vi "Read Config Unitest.vi"(8 "error in (no error)":errorcluster, 11 "main ref":T1) -> (0 "error out":errorcluster)   [LabVIEW 2025]
uses:
  v06/controls/LAB-IQ UI Data.ctl
  Traction Loop/Traction Receipe Enum.ctl
  Config file  FGV Unitest enum.ctl
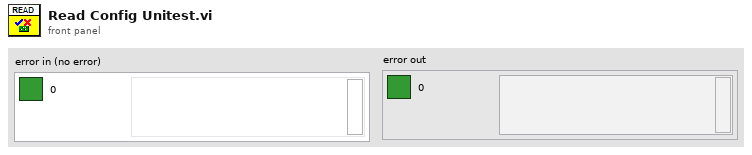
[diagram p1: front panel]
types:
  T1 = typedef "LAB-IQ UI Data.ctl" = cluster{"Main Home Screen":cluster{"GUI":refnum<vi>, "Platform Settings":refnum<vi>, "Configure":refnum<vi>, "Home":refnum<vi>, "EXIT":refnum<vi>, "service 2":refnum<vi>, "MainPage":refnum<vi>, "Analysis":refnum<vi>}, "Platform Settings":cluster{"mm/s  Surge":refnum<vi>, "Drive Error":refnum<vi>, "Disable Axis Jog Soft Limits":refnum<vi>, "mm/s  Sway":refnum<vi>, "Sway and Surge COM Status":refnum<vi>, "Heave COM Status":refnum<vi>, "Enable Platform":refnum<vi>, "Surge Forward Main":refnum<vi>, "Sway Right Main":refnum<vi>, "Sway Left Main":refnum<vi>, "Heave Down Main":refnum<vi>, "Heave Up main":refnum<vi>, "mm/s Heave":refnum<vi>, "mm/sec":refnum<vi>, "mm":refnum<vi>, "Surge Backward Main":refnum<vi>}, "Analysis Screen":cluster{"Analysis Home":refnum<vi>, "Surface Analysis":refnum<vi>, "Imaging":refnum<vi>, "Image Analysis":refnum<vi>, "Post Analysis":refnum<vi>}, "Config Screen":cluster{"Select Load Head":refnum<vi>, "Notes :":refnum<vi>, "FILE":refnum<vi>, "Sample ID :":refnum<vi>, "Operator ID :":refnum<vi>, "Operator Name :":refnum<vi>, "Auto":refnum<vi>}, "Motion Module":cluster{"zNL":refnum<vi>, "NL disp":refnum<vi>, "Rotary Tab":refnum<vi>, "Motion Direction:  3":refnum<vi>, "E.Velocity 2":refnum<vi>, "e.v/ssr 2":refnum<vi>, "Enter Fixed E.Velocity 2":refnum<vi>, "Enter Final SRR 2":refnum<vi>, "Enter initial SRR 2":refnum<vi>, "Enter Fixed SRR 2":refnum<vi>, "Enter the Final E.Velocity (m/s) 2":refnum<vi>, "Enter initial E.Velocity (m/s) 2":refnum<vi>, "Final Speed (RPM) 3":refnum<vi>, "Initial Speed (RPM) 2":refnum<vi>, "Enter the Final Velocity (m/s) 3":refnum<vi>, "Enter initial Velocity (m/s)  3":refnum<vi>, "Ramp Up 2":refnum<vi>, "TEST SELECTION":refnum<vi>, "SPEED SELECTION : ":refnum<vi>, "Angular Oscillation Set":refnum<vi>, "Traction":refnum<vi>, "Step Speed":refnum<vi>, "StepTable For Load-Speed":refnum<vi>, "StepTable For Speed":refnum<vi>, "Surge Forward MM":refnum<vi>, "Surge Backward MM":refnum<vi>, "M3 Image":refnum<vi>, "String 39":refnum<vi>, "Sway Left MM":refnum<vi>, "Sway Right MM":refnum<vi>, "Disable Axis Jog Soft Limits":refnum<vi>, "mm":refnum<vi>, "Heave Down MM":refnum<vi>, "Heave Up MM":refnum<vi>, "Wear Track Diameter (mm)":refnum<vi>, "Set WTD":refnum<vi>, "HomeScratch":refnum<vi>, "HomeRot":refnum<vi>, "PlaceModule":refnum<vi>, "Enter the Angle (Deg)":refnum<vi>, "Enter the Frequency (Hz)":refnum<vi>, "Motion Mode:":refnum<vi>, "LR Sway":refnum<vi>, "Rot Hor":refnum<vi>, "Scratch":refnum<vi>, "LR Cam":refnum<vi>, "MMBack":refnum<vi>, "MMNext":refnum<vi>, "Rot Ver":refnum<vi>, "Rotary Module Selection":refnum<vi>, "calculate rotary":refnum<vi>, "SPEED SELECTION : rotary":refnum<vi>, "Import 2":refnum<vi>, "Save 2":refnum<vi>, "File Path :  2":refnum<vi>, "String 45":refnum<vi>, "StepTable For Speed 3":refnum<vi>, "Enter the Speed(mm/sec)":refnum<vi>, "Enter the Speed(RPM)":refnum<vi>, "Enter Scratch Speed (mm/s):":refnum<vi>, "SwaySpeed Set":refnum<vi>, "Scartch Offset":refnum<vi>, "Motion type:":refnum<vi>, "HomeScratch 2":refnum<vi>, "Enter Scratch length (mm):":refnum<vi>, "Wear Track Diameter":refnum<vi>, "Rotary Speed Exced":refnum<vi>, "Scratch Mode":refnum<vi>, "No of Scratch":refnum<vi>}, "Environmental control":cluster{"Humidity  Status  3":refnum<vi>, "Low Temp  Status  2":refnum<vi>, "TK4 status 2":refnum<vi>, "Stage Temperature":refnum<vi>, "Sample Temperature":refnum<vi>, "Humidity (Amb)":refnum<vi>, "Clear List":refnum<vi>, "Add to list":refnum<vi>, "Wear":refnum<vi>, "Vibration":refnum<vi>, "Humidity (Chamber)":refnum<vi>, "Temperature (Chamber)":refnum<vi>, "ECR ":refnum<vi>, "Temperature (Amb)":refnum<vi>, "Microphone":refnum<vi>, "Acoustic Emission 3":refnum<vi>, "SNext":refnum<vi>, "APBack":refnum<vi>, "Enter the Temperature (°C):":refnum<vi>, "Enter the Stage \nTemperature (°C):":refnum<vi>, "Enter the Humidity (%Rh):":refnum<vi>, "Low Temp":refnum<vi>, "High Temp":refnum<vi>, "Humidity":refnum<vi>, "Sensors Picked":refnum<vi>}, "About Screen":cluster{"Password":refnum<vi>, "Home Service":refnum<vi>, "Advanced Setting":refnum<vi>, "About Tab":refnum<vi>, "ECR Port:":refnum<vi>, "Ramp Port:":refnum<vi>, "Installation/Replacement completed":refnum<vi>, "Loahead":refnum<vi>, "Heave and Surge COM Port:":refnum<vi>, "Sway COM Port:":refnum<vi>, "Temp Modbus:":refnum<vi>, "Humidity Port:":refnum<vi>, "Edit Gain Constants":refnum<vi>, "Save Gain Constants":refnum<vi>}, "Main Screen":cluster{"Main Screen Tab":refnum<vi>, "Angle and Frequency":refnum<vi>, "Stroke (mm)":refnum<vi>, "Angle (Deg)":refnum<vi>, "Main Speed Tab":refnum<vi>, "MTM MOTOR DISPLAY":refnum<vi>, "Disc Speed (m/sec)":refnum<vi>, "Ball Speed (m/sec)":refnum<vi>, "Disc Speed (RPM)":refnum<vi>, "Ball Speed (RPM)":refnum<vi>, "SPEED TAB":refnum<vi>, "Speed (m/sec)":refnum<vi>, "Set Speed (m/sec)":refnum<vi>, "Speed (RPM)":refnum<vi>, "Set Speed":refnum<vi>, "Time Tab":refnum<vi>, "Time ( HH:MM:SS ) 2":refnum<vi>, "Test Duration":refnum<vi>, "Test Duration 4":refnum<vi>, "TEST CYCLE":refnum<vi>, "TOTAL CYCLES":refnum<vi>, "Set Load (N)":refnum<vi>, "Temp Tabs":refnum<vi>, "Heater":refnum<vi>, "TK4 status":refnum<vi>, "ChamberTemp":refnum<vi>, "SetTmp":refnum<vi>, "Controller  Status":refnum<vi>, "ChamberTemp 2":refnum<vi>, "SetTmp 2":refnum<vi>, "Controller  Status 2":refnum<vi>, "ChamberTemp 3":refnum<vi>, "SetTmp 3":refnum<vi>, "Cooling":refnum<vi>, "Load Communication":refnum<vi>, "Ambient \nTemperature":refnum<vi>, "HumCOMStatus":refnum<vi>, "Ambient\n Humidity":refnum<vi>, "Freq (Hz)":refnum<vi>, "Load En":refnum<vi>, "NLt":refnum<vi>, "zNL 2":refnum<vi>, "Humidity On":refnum<vi>, "humidity disp":refnum<vi>, "Set Humidity":refnum<vi>, "NL disp 2":refnum<vi>, "Humidity On 2":refnum<vi>, "humidity disp 2":refnum<vi>, "Set Humidity 2":refnum<vi>, "NL disp 3":refnum<vi>, "AppLoadSeq scratch":refnum<vi>, "Stop Scratch":refnum<vi>, "ClrLog":refnum<vi>, "Trip Log":refnum<vi>, "STOP":refnum<vi>, "Start Test":refnum<vi>, "Test status":refnum<vi>, "AR Led":refnum<vi>, "Data":refnum<vi>, "Health":refnum<vi>, "Sway COM Status":refnum<vi>, "Heave COM Status":refnum<vi>, "Grp Tab":refnum<vi>, "Sub Graph":refnum<vi>, "SD (mm)":refnum<vi>, "Siliding distance Reset Graph":refnum<vi>, "SDGp":refnum<vi>, "Humidity Reset Graph":refnum<vi>, "HumrGp":refnum<vi>, "Acoustic Emission (mV)":refnum<vi>, "Aqucostic Reset Graph":refnum<vi>, "gACQUOS":refnum<vi>, "ECR RESET":refnum<vi>, "ECR":refnum<vi>, "Temperature Reset":refnum<vi>, "Acoustic Emission (mV) 2":refnum<vi>, "Aqucostic Reset Graph 2":refnum<vi>, "gACQUOS 2":refnum<vi>, "ECR RESET 2":refnum<vi>, "ECR 2":refnum<vi>, "Temperature Reset 2":refnum<vi>, "Temperature (deg c)":refnum<vi>, "Speed Reset Graph":refnum<vi>, "Speed Tab":refnum<vi>, "MTM DISC  SPEED":refnum<vi>, "MTM BALL SPEED":refnum<vi>, "speed mm/sec":refnum<vi>, "Hymidity":refnum<vi>, "Humidity Disable trip":refnum<vi>, "CoF Trip  2":refnum<vi>, "Depth Trip":refnum<vi>, "Weart Deapth":refnum<vi>, "Depth Reset Graph":refnum<vi>, "Weart":refnum<vi>, "Depthz":refnum<vi>, "Depth (µm)":refnum<vi>, "WearGp":refnum<vi>, "NL Trip 2":refnum<vi>, "Load pid":refnum<vi>, "Load Disable Trip":refnum<vi>, "Load Reset Graph":refnum<vi>, "NL Display 4":refnum<vi>, "Main Chart 3":refnum<vi>, "BACK":refnum<vi>, "Depth Trip 2":refnum<vi>, "COF TRIP ":refnum<vi>, "Friction Force (N)":refnum<vi>, "FF Reset Graph":refnum<vi>, "FF Disable Trip":refnum<vi>, "FF TRIP":refnum<vi>, "COF Disable Trip":refnum<vi>, "COF Reset Graph":refnum<vi>, "Start Test Temp":refnum<vi>, "zFF":refnum<vi>, "Friction Force (N) Graph":refnum<vi>, "Coefficient of Friction":refnum<vi>, "Scratch Start Test":refnum<vi>, "FF Tab":refnum<vi>, "Cyclic Friction Force (N)":refnum<vi>, "CZ FF":refnum<vi>, "Cyclic Friction Force (N) Graph":refnum<vi>, "Cyclic Coefficient of Friction":refnum<vi>, "Cyclic FF TRIP":refnum<vi>, "Cyclic FF Disable Trip":refnum<vi>, "cyclic COF Disable Trip":refnum<vi>, "cyclic COF TRIP":refnum<vi>, "cyclic COF Reset Graph":refnum<vi>, "Cyclic FF Reset Graph":refnum<vi>, "Test Trip":refnum<vi>, "Multi Scratch Pass":refnum<vi>, "Scratch Start Recording":refnum<vi>, "Coefficient of Friction 2":refnum<vi>, "Acoustic Emission":refnum<vi>, "Friction Force (N) 2":refnum<vi>, "Depth (Microns)":refnum<vi>, "Normal Load ( N )":refnum<vi>}, "Loading":cluster{"Indentation":refnum<vi>, "Reference Sample":refnum<vi>, "Load Cell Communication Slide":refnum<vi>, "com 3":refnum<vi>, "com":refnum<vi>, "DecaForce COM Status":refnum<vi>, "Update":refnum<vi>, "Clear 3":refnum<vi>, "seq":refnum<vi>, "Stribeck table":refnum<vi>, "Stribeck Table  For loading":refnum<vi>, "Loading Mode":refnum<vi>, "Enter the Final Load (N)":refnum<vi>, "Enter the CoF Trip":refnum<vi>, "Enter the Friction Force Trip":refnum<vi>, "Enter the Normal load Trip":refnum<vi>, "Enter the Load  (N)":refnum<vi>, "KiloForce":refnum<vi>, "DecaForce ":refnum<vi>, "MicroForce":refnum<vi>, "LHBack":refnum<vi>, "LHNext":refnum<vi>, "Enter the Loading Rate (N/min)":refnum<vi>, "Message":refnum<vi>, "Warning 2":refnum<vi>, "SSP 0.75":refnum<vi>, "SSP 0.5":refnum<vi>, "SSP 0.3":refnum<vi>, "Warning":refnum<vi>, "gui GIF":refnum<vi>, "Communication is established":refnum<vi>, "AppLoad 4":refnum<vi>, "Multipoint":refnum<vi>, "Load Selection":refnum<vi>}, "PID":cluster{"Ramp":refnum<vi>, "Vertical load (N)":refnum<vi>, "apply load":refnum<vi>, "apply load 2":refnum<vi>, "Enter ByPass Load":refnum<vi>, "Bypass Load":refnum<vi>, "gFF Rot":refnum<vi>}, "Config Parameters":cluster{"Tab Control 3":refnum<vi>, "Tab Control 19":refnum<vi>, "SAMPLES":refnum<vi>, "Re-initilaize":refnum<vi>, "Filter ON/OFF":refnum<vi>, "TracHomeSurgeOffsetCounts 10MM":refnum<vi>, "TracHomeSwayOffsetCounts 10MM":refnum<vi>, "Acoustic Emission:":refnum<vi>, "Apply Filter (FF)":refnum<vi>, "Filter% 2":refnum<vi>, "Apply Filter (Load)":refnum<vi>, "Filter% ":refnum<vi>, "Sway distance (mm)":refnum<vi>, "Surge distance (mm)":refnum<vi>, "DataSavingLoopDelay(ms)":refnum<vi>, "SAVE 2":refnum<vi>, "Enter Distance":refnum<vi>, "Sway Counts:":refnum<vi>, "Distance (mm): 3":refnum<vi>, "Surge Counts:":refnum<vi>, "Distance (mm): 2":refnum<vi>, "Distance (mm):":refnum<vi>, "Heave Counts:":refnum<vi>, "LRMHomeSurgeOffsetCounts":refnum<vi>, "LRMHomeSwayOffsetCounts":refnum<vi>, "TracHomeSurgeOffsetCounts 20MM":refnum<vi>, "TracHomeSwayOffsetCounts 20MM":refnum<vi>, "RotHomeSwayOffsetCounts":refnum<vi>, "RotHomeSurgeOffsetCounts":refnum<vi>, "Heave distance":refnum<vi>, "Zmm":refnum<vi>, "Heave Pulses/mm":refnum<vi>, "Surge Pulses/mm":refnum<vi>, "Sway Pulses/mm":refnum<vi>, "Heave Pitch":refnum<vi>, "Surge Pitch":refnum<vi>, "Sway Pitch":refnum<vi>, "Heave PPR":refnum<vi>, "Surge PPR":refnum<vi>, "Sway PPR":refnum<vi>, "Tab Control 5":refnum<vi>, "Tab Control 14":refnum<vi>, "Tab Control 26":refnum<vi>, "AE":refnum<vi>, "Heave Loop Delay":refnum<vi>, "Heave PID Speed":refnum<vi>, "Surge Jog Speed":refnum<vi>, "Heave Jog Speed":refnum<vi>, "Sway Loop Delay":refnum<vi>, "Sway PID Speed":refnum<vi>, "Sway Jog Speed":refnum<vi>, "DEPTH TRIP VALUE":refnum<vi>, "LOAD TRIP VALUE":refnum<vi>, "DEPTH TRIP   ENABLE":refnum<vi>, "LOAD TRIP  ENABLE":refnum<vi>, "CYCLIC FF TRIP VALUE":refnum<vi>, "FF TRIP VALUE":refnum<vi>, "CYCLIC CoF TRIP VALUE":refnum<vi>, "COF TRIP VALUE":refnum<vi>, "CYCLIC COF TRIP  ENABLE":refnum<vi>, "CYCLIC FF TRIP  ENABLE":refnum<vi>, "FF TRIP  ENABLE":refnum<vi>, "COF TRIP  ENABLE":refnum<vi>, "JOG TRIP LOAD VALUE (N)":refnum<vi>, "Rotary Vertical":refnum<vi>, "Traction":refnum<vi>, "Scratch":refnum<vi>, "LRM CAM":refnum<vi>, "Sway LRM":refnum<vi>, "Rotary Horizontal":refnum<vi>, "SURGE SPEED":refnum<vi>, "SURGE BACKWARD COUNT":refnum<vi>, "SURGE FORWARD COUNT":refnum<vi>, "Start Button":refnum<vi>}, "Loading Com Port":cluster{"ClearAll":refnum<vi>, "Mz(Nm)":refnum<vi>, "My(Nm)":refnum<vi>, "Mx(Nm)":refnum<vi>, "Save Dwell":refnum<vi>, "Acq Delay (ms)":refnum<vi>, "Burst Delay (ms)":refnum<vi>, "model":refnum<vi>, "SN":refnum<vi>, "FFx(N)":refnum<vi>, "Sensor IP":refnum<vi>, "Port":refnum<vi>, "FFy(N)":refnum<vi>, "Load(N)":refnum<vi>, "delete Handle":refnum<vi>, "Create Handle":refnum<vi>, "ft_data":refnum<vi>, "ft_range":refnum<vi>, "ft_data 2":refnum<vi>, "stop 6":refnum<vi>, "running_flag":refnum<vi>, "ft_udp_handle":refnum<vi>, "get-data-return":refnum<vi>, "get-range-return":refnum<vi>, "zero-return":refnum<vi>, "filter-return":refnum<vi>, "initial-return":refnum<vi>, "deleteHandle-result":refnum<vi>, "Load Cell Temp":refnum<vi>, "Load Cell":refnum<vi>, "ZeroAll":refnum<vi>, "FORCE (N)":refnum<vi>, "TORQUE (N-m)":refnum<vi>, "Load Cell Link":refnum<vi>}, "Heave AND Surge":cluster{"SURGE POSE":refnum<vi>, "error out Read":refnum<vi>, "HEAVE POSE":refnum<vi>, "State":refnum<vi>, "Homed":refnum<vi>, "Sequence ID":refnum<vi>, "error out Write":refnum<vi>, "faultCode":refnum<vi>, "Ack ID":refnum<vi>, "SPEED":refnum<vi>, "Distance":refnum<vi>, "Mode Command":refnum<vi>, "Heave and Surge Read":refnum<vi>, "Read Heave Temp":refnum<vi>, "Spare 15":refnum<vi>, "Spare 14":refnum<vi>, "Spare 13":refnum<vi>, "Spare 12":refnum<vi>, "Spare 11":refnum<vi>, "Spare 10":refnum<vi>, "Spare 9":refnum<vi>, "Spare 8":refnum<vi>, "Spare 7":refnum<vi>, "Spare 4":refnum<vi>, "Spare 3":refnum<vi>, "Spare 2":refnum<vi>, "Humidity":refnum<vi>, "Temp":refnum<vi>, "Node Id":refnum<vi>, "Spare 1":refnum<vi>, "SPARE 4":refnum<vi>, "SPARE 3":refnum<vi>, "SPARE 2":refnum<vi>, "SPARE 1":refnum<vi>, "fwMajor":refnum<vi>, "fwMinor":refnum<vi>, "Manual Write":refnum<vi>, "Heave and Surge Write":refnum<vi>, "SPARE 5":refnum<vi>, "Reserved ":refnum<vi>, "SPARE 8":refnum<vi>, "SPARE 6":refnum<vi>, "SPARE 7":refnum<vi>, "SPARE 17":refnum<vi>, "SPARE 16":refnum<vi>, "SPARE 15":refnum<vi>, "SPARE 14":refnum<vi>, "SPARE 13":refnum<vi>, "SPARE 12":refnum<vi>, "SPARE 11":refnum<vi>, "SPARE 10":refnum<vi>, "SPARE 9":refnum<vi>, "System UPTIME":refnum<vi>, "Missed Packets":refnum<vi>, "faultCode Surge Right":refnum<vi>, "faultCode Surge Left":refnum<vi>, "faultCode Heave":refnum<vi>, "UPLINK HEAVE":refnum<vi>, "DOWNLINK HEAVE":refnum<vi>}, "New PID LOGIC":cluster{"Fine Tune Zone":refnum<vi>, "PID SDelay":refnum<vi>, "Max_pos_limit":refnum<vi>, "Min_pos_limit":refnum<vi>, "i_limit":refnum<vi>, "pct_scale":refnum<vi>, "Deadband":refnum<vi>, "Kd":refnum<vi>, "Ki":refnum<vi>, "Kp":refnum<vi>, "Current Position":refnum<vi>, "Set Load":refnum<vi>, "Current Load":refnum<vi>, "Pulse delta":refnum<vi>, "Init Step":refnum<vi>, "Max Step Linit":refnum<vi>, "min_deadband_floor":refnum<vi>, "dynamic_spindle_noise_scalar":refnum<vi>, "min_finetune_floor":refnum<vi>, "filter_alpha":refnum<vi>, "PID":refnum<vi>}, "SWAY ":cluster{"fwMajor":refnum<vi>, "Homed":refnum<vi>, "Rotary POSE":refnum<vi>, "State":refnum<vi>, "SWAY POSE":refnum<vi>, "Ack ID":refnum<vi>, "faultCode":refnum<vi>, "Node Id":refnum<vi>, "fwMinor":refnum<vi>, "Spare 6":refnum<vi>, "Spare 5":refnum<vi>, "Spare 4":refnum<vi>, "Spare 3":refnum<vi>, "Spare 2":refnum<vi>, "Spare 1":refnum<vi>, "Spare 7":refnum<vi>, "SPARE  5":refnum<vi>, "error out Write  SWAY ":refnum<vi>, "error out Read SWAY ":refnum<vi>, "Manual Write SWAY ":refnum<vi>, "SWAY WRITE":refnum<vi>, "SPARE  4":refnum<vi>, "SPARE  3":refnum<vi>, "SPARE 2":refnum<vi>, "SPARE 1":refnum<vi>, "Spare 15":refnum<vi>, "Spare 14":refnum<vi>, "Spare 13":refnum<vi>, "Spare 12":refnum<vi>, "Spare 11":refnum<vi>, "Spare 9":refnum<vi>, "Spare 8":refnum<vi>, "SPEED":refnum<vi>, "Distance":refnum<vi>, "Mode Command":refnum<vi>, "Sequence ID":refnum<vi>, "SWAY READ":refnum<vi>, "Spare 10":refnum<vi>, "Read SWAY Temp":refnum<vi>, "faultCode Sway ":refnum<vi>, "Missed Packets":refnum<vi>, "System UPTIME sway":refnum<vi>, "SPARE 6":refnum<vi>, "SPARE 7":refnum<vi>, "SPARE 9":refnum<vi>, "SPARE 11":refnum<vi>, "SPARE 10":refnum<vi>, "SPARE 8":refnum<vi>, "SPARE 13":refnum<vi>, "SPARE 12":refnum<vi>, "SPARE 17":refnum<vi>, "SPARE 16":refnum<vi>, "SPARE 15":refnum<vi>, "SPARE 14":refnum<vi>, "Reserved":refnum<vi>, "faultCode Rotary":refnum<vi>, "UPLINK SWAY":refnum<vi>, "DOWNLINK SWAY":refnum<vi>}, "Analysis Screen":cluster{"Analysis Home":refnum<vi>, "Refresh 2":refnum<vi>, "MEAN 4":refnum<vi>, "SD 4":refnum<vi>, "VARIANCE 4":refnum<vi>, "MEAN  3":refnum<vi>, "SD  3":refnum<vi>, "VARIANCE  3":refnum<vi>, "MEAN 2":refnum<vi>, "SD  2":refnum<vi>, "VARIANCE 2":refnum<vi>, "MEAN":refnum<vi>, "SD":refnum<vi>, "VARIANCE":refnum<vi>, "File 4 Discription":refnum<vi>, "OPEN 4":refnum<vi>, "File Name 4":refnum<vi>, "OPEN 3":refnum<vi>, "File 3 Discription":refnum<vi>, "File Name 3":refnum<vi>, "Y-AXIS":refnum<vi>, "X-AXIS":refnum<vi>, "XY Graph":refnum<vi>, "File Name 2":refnum<vi>, "File Name 1":refnum<vi>, "OPEN 2":refnum<vi>, "OPEN 1":refnum<vi>, "File 1 Discription ":refnum<vi>, "File 2 Discription":refnum<vi>, "Export":refnum<vi>, "File Format":refnum<vi>}, "Traction":cluster{"faultCode Traction 2":refnum<vi>, "faultCode Traction 1":refnum<vi>, "Missed Packets":refnum<vi>, "System UPTIME Traction":refnum<vi>, "SPARE 17":refnum<vi>, "SPARE 16":refnum<vi>, "SPARE 15":refnum<vi>, "SPARE 14":refnum<vi>, "SPARE 13":refnum<vi>, "SPARE 12":refnum<vi>, "SPARE 11":refnum<vi>, "SPARE 10":refnum<vi>, "SPARE 9":refnum<vi>, "SPARE 8":refnum<vi>, "SPARE 7":refnum<vi>, "SPARE 6":refnum<vi>, "Reserved":refnum<vi>, "SPARE  5":refnum<vi>, "Manual Write TRACTION":refnum<vi>, "TRACTION WRITE":refnum<vi>, "SPARE  4":refnum<vi>, "SPARE  3":refnum<vi>, "SPARE 2":refnum<vi>, "SPARE 1":refnum<vi>, "Spare 7":refnum<vi>, "Spare 6":refnum<vi>, "Spare 5":refnum<vi>, "Spare 4":refnum<vi>, "Spare 2":refnum<vi>, "Spare 1":refnum<vi>, "Node Id":refnum<vi>, "Read TRACTION Temp":refnum<vi>, "fwMinor":refnum<vi>, "fwMajor":refnum<vi>, "faultCode":refnum<vi>, "TRACTION POSE":refnum<vi>, "TRACTION POSE 2":refnum<vi>, "Homed":refnum<vi>, "State":refnum<vi>, "Ack ID":refnum<vi>, "SPEED":refnum<vi>, "Distance":refnum<vi>, "Mode Command":refnum<vi>, "Sequence ID":refnum<vi>, "error out Read TRACTION":refnum<vi>, "error out Write  TRACTION":refnum<vi>, "TRACTION READ":refnum<vi>, "Spare 3":refnum<vi>, "Downlink traction":refnum<vi>, "Uplink Traction":refnum<vi>}, "Traction reciepe":cluster{"SRR Sweep Range (%) Stribeck":refnum<vi>, "Traction Receipe":refnum<vi>, "Total Execution Time":refnum<vi>, "Total Steps":refnum<vi>, "Duration / Step (s)  Stribeck":refnum<vi>, "STRIBECK Fixed SRR List (%)":refnum<vi>, "Duration / Step (s) Traction":refnum<vi>, "SRR Sweep Range (%) traction":refnum<vi>, "Rolling Speed (mm/s)":refnum<vi>, "Temperature Stages (°C)":refnum<vi>, "Ball Load (N)":refnum<vi>, "Lubricant Name":refnum<vi>, "Profile File Name":refnum<vi>, "SET entrainment Velocity":refnum<vi>, "Test Array Size":refnum<vi>, "SRR INDEX [ STRIBECK]":refnum<vi>, "Stribeck Size":refnum<vi>, "SET SRR":refnum<vi>, "ELAPSED TIMER ":refnum<vi>, "BALL SET RPM":refnum<vi>, "DISC SET RPM":refnum<vi>, "SET LOAD":refnum<vi>, "TEMPERATURE READ":refnum<vi>, "SET TEMPERATURE":refnum<vi>, "Traction Size":refnum<vi>, "DISC SPEED (rpm)":refnum<vi>, "BALL SPEED (rpm)":refnum<vi>, "BALL WEAR TRACK":refnum<vi>, "DISC WEARTRACK":refnum<vi>, "SRR INDEX [ TRACTION]":refnum<vi>, "Start Index Type":refnum<vi>, "Enum - Menu":refnum<vi>, "Ball (mm/sec)":refnum<vi>, "Disc (mm/sec)":refnum<vi>, "Traction Receipe Update Details":refnum<vi>}, "Traction Control":cluster{"HomeTraction":refnum<vi>, "Demo Mode Display":refnum<vi>, "Traction Message":refnum<vi>, "Traction Step Update Details":refnum<vi>, "Main Tab sequence for selection":refnum<vi>, "Ramp Tab":refnum<vi>, "e.v/ssr":refnum<vi>, "Enter Fixed E.Velocity":refnum<vi>, "Enter Final SRR":refnum<vi>, "Enter initial SRR":refnum<vi>, "Enter Fixed SRR":refnum<vi>, "Enter the Final E.Velocity (m/s)":refnum<vi>, "Enter initial E.Velocity (m/s)":refnum<vi>, "Ball WTD":refnum<vi>, "E.Velocity":refnum<vi>, "Enter the Final Velocity (m/s)":refnum<vi>, "Enter initial Velocity (m/s)":refnum<vi>, "Ramp Up   Disc":refnum<vi>, "Initial DiscSpeed (RPM)":refnum<vi>, "Final Speed (RPM) Ball":refnum<vi>, "Final Speed (RPM)":refnum<vi>, "Initial Speed (RPM) Ball":refnum<vi>, "Enter the Final Velocity (m/s) Ball":refnum<vi>, "Enter initial Velocity (m/s) Ball":refnum<vi>, "Ramp Up":refnum<vi>, "ExceedBallSpeed step":refnum<vi>, "ExceedDiscSpeed":refnum<vi>, "BallSpeed Exceed Indication":refnum<vi>, "Apply":refnum<vi>, "SPEED SELECTION : MTM":refnum<vi>, "SPEED SELECTION : MTM 2":refnum<vi>, "TEST SELECTION (MTM)":refnum<vi>, "MTM Test Selection":refnum<vi>, "File Path Tab":refnum<vi>, "File Path String":refnum<vi>, "Save":refnum<vi>, "Save  2":refnum<vi>, "Import ":refnum<vi>, "File Path :":refnum<vi>, "Step Sequence Indication Tab":refnum<vi>, "Step Sequence Indication":refnum<vi>, "Calculate Step":refnum<vi>, "StepTable":refnum<vi>, "ExceedDiscSpeed  Cinstant Speed":refnum<vi>, "ExceedBallSpeed Constant":refnum<vi>, "TEST SELECTION (MTM) 2":refnum<vi>, "SPEED SELECTION : MTM 3":refnum<vi>, "MTM Test Selection 2":refnum<vi>, "Enter the Speed (m/sec): ":refnum<vi>, "Enter the Speed (m/sec):  2":refnum<vi>, "Enter the Speed (RPM):":refnum<vi>, "Lower Spped ":refnum<vi>, "Upper":refnum<vi>, "Enter the Speed (RPM):Ball":refnum<vi>, "Disc Motion Direction: ":refnum<vi>, "Ball Motion Direction :":refnum<vi>, "Motion Mode: ":refnum<vi>, "Wear Track Diameter (mm) ":refnum<vi>, "Disc Speed Indicator":refnum<vi>, "ExceedBallSpeed":refnum<vi>}, "Acquostic":cluster{"Last Config Rejected ":refnum<vi>, "rx command count":refnum<vi>, "Current Filter Id":refnum<vi>, "Isolated Gain":refnum<vi>, "DAQ Status":refnum<vi>, "error out":refnum<vi>, "error in (no error)":refnum<vi>, "Uplink Packet":refnum<vi>, "data out":refnum<vi>, "Downlink Packet":refnum<vi>, "Gains":refnum<vi>, "Manual Write Acquostic":refnum<vi>, "Acoustic Graphs":refnum<vi>}, "ABOUT":cluster{"version":refnum<vi>, "Operating System":refnum<vi>, "Version":refnum<vi>, "Workorder":refnum<vi>, "Runtime":refnum<vi>, "Instrument Serial":refnum<vi>, "Firmware Version":refnum<vi>, "Info":refnum<vi>}, "Temperature Port":cluster{"Temperature":refnum<vi>, "error out Temperature":refnum<vi>, "READ TEMPERATURE":refnum<vi>}}
  T2 = typedef "Config file  FGV Unitest enum.ctl" = enum16{"OPEN", "READ", "WRITE", "CLOSE"}
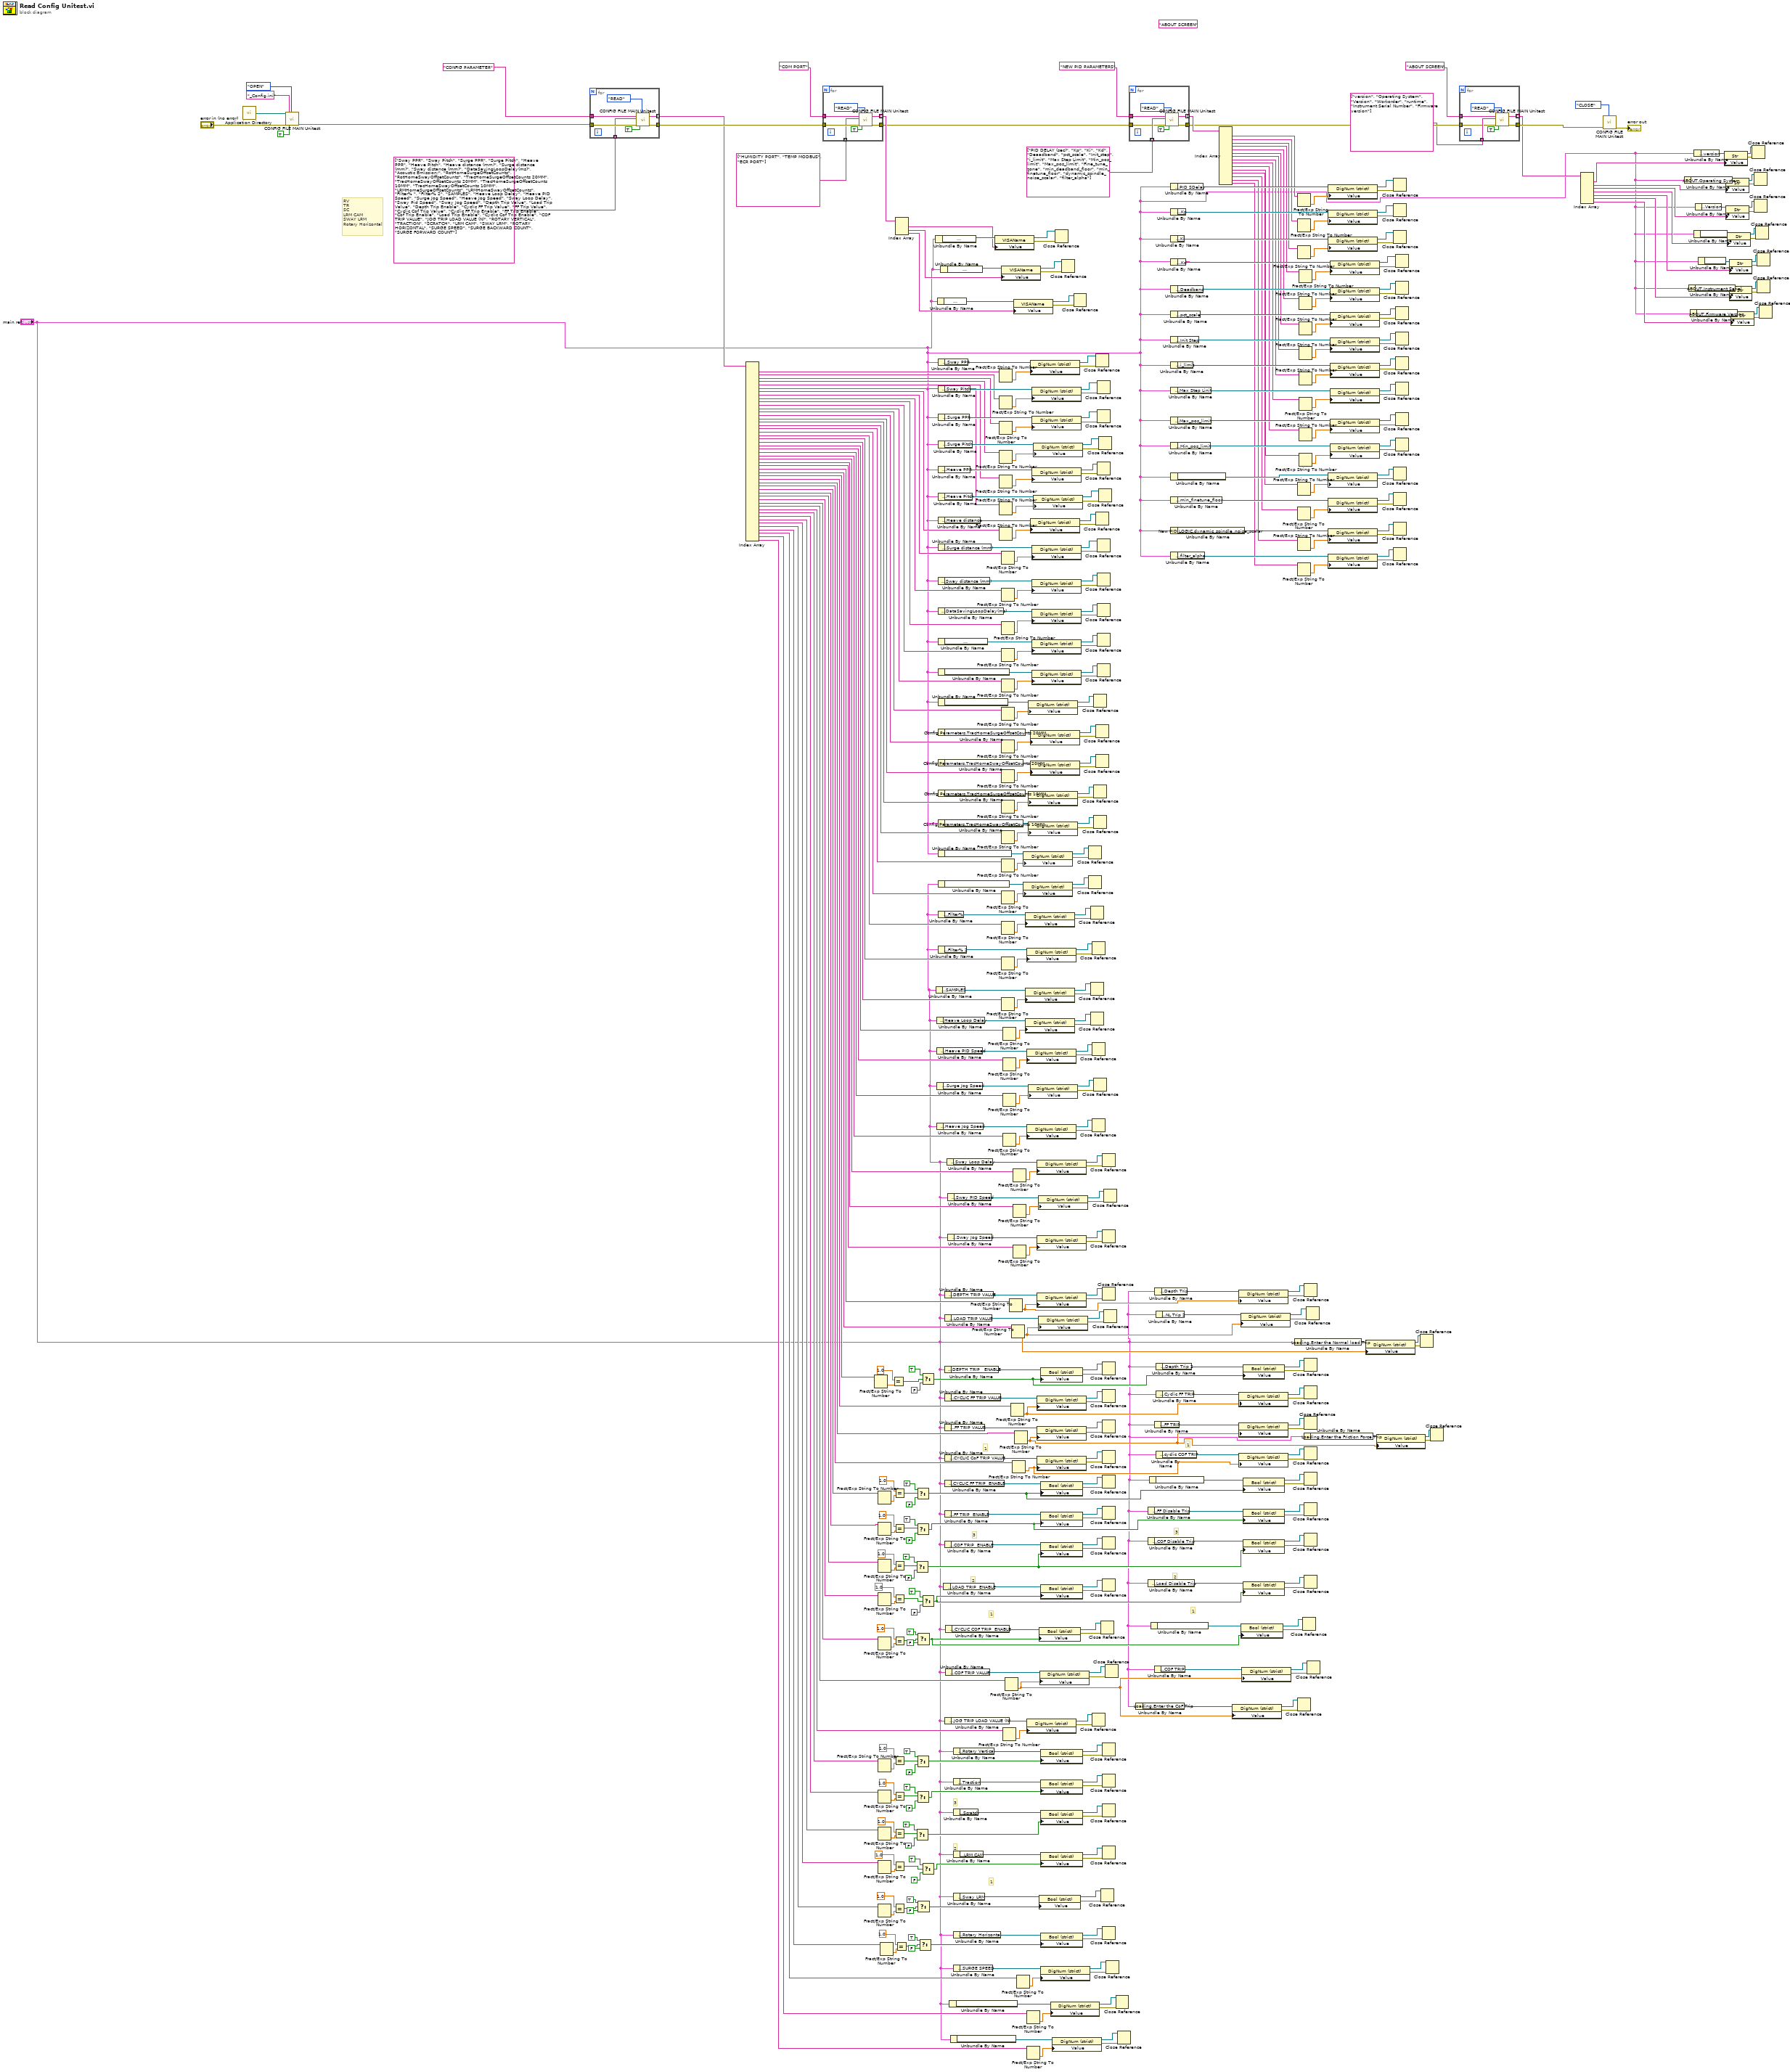
[diagram p0: block diagram]
diagram:
  (unwired) "ABOUT SCREEN" ("WRITE /READ SECTION")
  # "RV\nTR\nSC\nLRM CAM\nSWAY LRM\nRotary Horizontal"
  # "3"
  # "2"
  # "1"
  # "3"
  # "2"
  # "1"
  # "1"
  # "3"
  # "2"
  # "1"
  # "1"
  n1 = call <vilib>:"Application Directory.vi"() -> ("Application Directory"=w496:path)
  n2 = call "CONFIG FILE MAIN Unitest.vi"("File Path"=w496, "error in"="error in (no error)", "file name"="_Config.ini", "PARAMETER/CONFIG"=TRUE, "Config Enum"=Config_file__FGV_Unitest_enum."OPEN") -> ("error out"=w495:errorcluster)  [unwired: 13 in, 1 out]
  n3 = for {
    tunnel: w495 -> [w507]
    tunnel: "CONFIG PARAMETER" ("WRITE /READ SECTION") -> [w506]
    tunnel: [w505] -> w493
    tunnel: [w502] -> w414 mode=indexing
    tunnel: string[] ["Sway PPR", "Sway Pitch", "Surge PPR", "Surge Pitch", "Heave PPR", "Heave Pitch", "Heave distance (mm)", "Surge distance (mm)", "Sway distance (mm)", "DataSavingLoopDelay(ms)", "Acoustic Emission:", "RotHomeSurgeOffsetCounts", "RotHomeSwayOffsetCounts", "TracHomeSurgeOffsetCounts 20MM", "TracHomeSwayOffsetCounts 20MM", "TracHomeSurgeOffsetCounts 10MM", "TracHomeSwayOffsetCounts 10MM", "LRMHomeSurgeOffsetCounts", "LRMHomeSwayOffsetCounts", "Filter% ", "Filter% 2", "SAMPLES", "Heave Loop Delay", "Heave PID Speed", "Surge Jog Speed", "Heave Jog Speed", "Sway Loop Delay", "Sway Pid Speed", "Sway Jog Speed", "Depth Trip Value", "Load Trip Value", "Depth Trip Enable", "Cyclic FF Trip Value", "FF Trip Value", "Cyclic Cof Trip Value", "Cyclic FF Trip Enable", "FF Trip Enable", "Cof Trip Enable", "Load Trip Enable", "Cyclic Cof Trip Enable", "COF TRIP VALUE", "JOG TRIP LOAD VALUE (N)", "ROTARY VERTICAL", "TRACTION", "SCRATCH", "LRM CAM", "SWAY LRM", "ROTARY HORIZONTAL", "SURGE SPEED", "SURGE BACKWARD COUNT", "SURGE FORWARD COUNT"] -> [w501] mode=indexing
    n4 = call "CONFIG FILE MAIN Unitest.vi"("WRITE /READ SECTION"=w506, "READ KEY"=w501, "error in"=w507, "PARAMETER/CONFIG"=TRUE, "Config Enum"=Config_file__FGV_Unitest_enum."READ") -> ("READ VALUE"=w502:string, "error out"=w505:errorcluster)  [unwired: 13 in]
  }
  n5 = Index Array(array=w414) -> (element #1=w413:string, element #2=w412:string, element #3=w411:string, element #4=w410:string, element #5=w409:string, element #6=w408:string, element #7=w407:string, element #8=w406:string, element #9=w405:string, element #10=w404:string, element #11=w403:string, element #12=w402:string, element #13=w401:string, element #14=w400:string, element #15=w399:string, element #16=w398:string, element #17=w397:string, element #18=w396:string, element #19=w395:string, element #20=w394:string, element #21=w393:string, element #22=w392:string, element #23=w353:string, element #24=w352:string, element #25=w351:string, element #26=w350:string, element #27=w279:string, element #28=w278:string, element #29=w277:string, element #30=w227:string, element #31=w226:string, element #32=w225:string, element #33=w224:string, element #34=w223:string, element #35=w222:string, element #36=w221:string, element #37=w220:string, element #38=w219:string, element #39=w218:string, element #40=w217:string, element #41=w163:string, element #42=w116:string, element #43=w61:string, element #44=w60:string, element #45=w59:string, element #46=w58:string, element #47=w57:string, element #48=w56:string, element #49=w42:string, element #50=w41:string, element #51=w40:string)  [unwired: 51 in]
  n6 = for {
    tunnel: w493 -> [w514]
    tunnel: "COM PORT" ("WRITE /READ SECTION") -> [w513]
    tunnel: [w512] -> w348
    tunnel: string[] ["HUMIDITY PORT", "TEMP MODBUS", "ECR PORT"] -> [w509] mode=indexing
    tunnel: [w508] -> w416 mode=indexing
    n7 = call "CONFIG FILE MAIN Unitest.vi"("WRITE /READ SECTION"=w513, "READ KEY"=w509, "error in"=w514, "PARAMETER/CONFIG"=TRUE, "Config Enum"=Config_file__FGV_Unitest_enum."READ") -> ("READ VALUE"=w508:string, "error out"=w512:errorcluster)  [unwired: 13 in]
  }
  n8 = Fract/Exp String To Number(string=w225) -> (number=w239:dbl)  [unwired: 3 in, 1 out]
  n9 = Fract/Exp String To Number(string=w221) -> (number=w240:dbl)  [unwired: 3 in, 1 out]
  n10 = Fract/Exp String To Number(string=w220) -> (number=w238:dbl)  [unwired: 3 in, 1 out]
  n11 = Fract/Exp String To Number(string=w219) -> (number=w237:dbl)  [unwired: 3 in, 1 out]
  n12 = Fract/Exp String To Number(string=w218) -> (number=w236:dbl)  [unwired: 3 in, 1 out]
  n13 = Fract/Exp String To Number(string=w217) -> (number=w235:dbl)  [unwired: 3 in, 1 out]
  n14 = Fract/Exp String To Number(string=w61) -> (number=w86:dbl)  [unwired: 3 in, 1 out]
  n15 = Fract/Exp String To Number(string=w60) -> (number=w87:dbl)  [unwired: 3 in, 1 out]
  n16 = Fract/Exp String To Number(string=w59) -> (number=w88:dbl)  [unwired: 3 in, 1 out]
  n17 = Fract/Exp String To Number(string=w58) -> (number=w89:dbl)  [unwired: 3 in, 1 out]
  n18 = Fract/Exp String To Number(string=w57) -> (number=w90:dbl)  [unwired: 3 in, 1 out]
  n19 = Fract/Exp String To Number(string=w56) -> (number=w67:dbl)  [unwired: 3 in, 1 out]
  n20 = Equal?(x=1.0, y=w239) -> (x = y?=w200:bool)
  n21 = Equal?(x=1.0, y=w240) -> (x = y?=w203:bool)
  n22 = Equal?(x=1.0, y=w238) -> (x = y?=w204:bool)
  n23 = Equal?(x=1.0, y=w237) -> (x = y?=w205:bool)
  n24 = Equal?(x=1.0, y=w236) -> (x = y?=w206:bool)
  n25 = Equal?(x=1.0, y=w235) -> (x = y?=w228:bool)
  n26 = Equal?(x=1.0, y=w86) -> (x = y?=w110:bool)
  n27 = Equal?(x=1.0, y=w87) -> (x = y?=w109:bool)
  n28 = Equal?(x=1.0, y=w88) -> (x = y?=w108:bool)
  n29 = Equal?(x=1.0, y=w89) -> (x = y?=w107:bool)
  n30 = Equal?(x=1.0, y=w90) -> (x = y?=w96:bool)
  n31 = Index Array(array=w416) -> (element #1=w1:string, element #2=w415:string, element #3=w6:string)  [unwired: 3 in]
  n32 = Equal?(x=1.0, y=w67) -> (x = y?=w65:bool)
  n33 = Select(t=TRUE, s=w205, f=FALSE) -> (s? t:f=w160:bool)
  n34 = Select(t=TRUE, s=w108, f=FALSE) -> (s? t:f=w113:bool)
  n35 = Select(t=TRUE, s=w203, f=FALSE) -> (s? t:f=w158:bool)
  n36 = Select(t=TRUE, s=w204, f=FALSE) -> (s? t:f=w159:bool)
  n37 = Select(t=TRUE, s=w110, f=FALSE) -> (s? t:f=w115:bool)
  n38 = Select(t=TRUE, s=w109, f=FALSE) -> (s? t:f=w114:bool)
  n39 = Select(t=TRUE, s=w228, f=FALSE) -> (s? t:f=w162:bool)
  n40 = Select(t=TRUE, s=w96, f=FALSE) -> (s? t:f=w111:bool)
  n41 = Select(t=TRUE, s=w65, f=FALSE) -> (s? t:f=w62:bool)
  n42 = Select(t=TRUE, s=w200, f=FALSE) -> (s? t:f=w155:bool)
  n43 = Select(t=TRUE, s=w206, f=FALSE) -> (s? t:f=w161:bool)
  n44 = Select(t=TRUE, s=w107, f=FALSE) -> (s? t:f=w112:bool)
  n45 = Unbundle By Name("main ref") -> ("About Screen.Humidity Port:"=w5:refnum<vi>)
  n46 = Unbundle By Name("main ref") -> ("Config Parameters.SAMPLES"=w428:refnum<vi>)
  n47 = Unbundle By Name("main ref") -> ("Config Parameters.Heave Loop Delay"=w356:refnum<vi>)
  n48 = Unbundle By Name("main ref") -> ("Config Parameters.Heave PID Speed"=w357:refnum<vi>)
  n49 = Unbundle By Name("main ref") -> ("Config Parameters.Surge Jog Speed"=w361:refnum<vi>)
  n50 = Unbundle By Name("main ref") -> ("Config Parameters.Heave Jog Speed"=w362:refnum<vi>)
  n51 = Unbundle By Name("main ref") -> ("About Screen.ECR Port:"=w418:refnum<vi>)
  n52 = Unbundle By Name("main ref") -> ("Config Parameters.Sway PPR"=w489:refnum<vi>)
  n53 = Unbundle By Name("main ref") -> ("Config Parameters.Sway Pitch"=w484:refnum<vi>)
  n54 = Unbundle By Name("main ref") -> ("Config Parameters.Surge PPR"=w478:refnum<vi>)
  n55 = Unbundle By Name("main ref") -> ("Config Parameters.Surge Pitch"=w483:refnum<vi>)
  n56 = Unbundle By Name("main ref") -> ("Config Parameters.Heave PPR"=w477:refnum<vi>)
  n57 = Unbundle By Name("main ref") -> ("Config Parameters.Heave Pitch"=w473:refnum<vi>)
  n58 = Unbundle By Name("main ref") -> ("Config Parameters.Heave distance"=w467:refnum<vi>)
  n59 = Unbundle By Name("main ref") -> ("Config Parameters.Surge distance (mm)"=w471:refnum<vi>)
  n60 = Unbundle By Name("main ref") -> ("Config Parameters.Sway distance (mm)"=w465:refnum<vi>)
  n61 = Unbundle By Name("main ref") -> ("Config Parameters.DataSavingLoopDelay(ms)"=w462:refnum<vi>)
  n62 = Unbundle By Name("main ref") -> ("Config Parameters.Acoustic Emission:"=w459:refnum<vi>)
  n63 = Unbundle By Name("main ref") -> ("Config Parameters.RotHomeSurgeOffsetCounts"=w456:refnum<vi>)
  n64 = Unbundle By Name("main ref") -> ("Config Parameters.RotHomeSwayOffsetCounts"=w453:refnum<vi>)
  n65 = Unbundle By Name("main ref") -> ("Config Parameters.TracHomeSurgeOffsetCounts 20MM"=w450:refnum<vi>)
  n66 = Unbundle By Name("main ref") -> ("Config Parameters.TracHomeSwayOffsetCounts 20MM"=w447:refnum<vi>)
  n67 = Unbundle By Name("main ref") -> ("Config Parameters.TracHomeSurgeOffsetCounts 10MM"=w443:refnum<vi>)
  n68 = Unbundle By Name("main ref") -> ("Config Parameters.TracHomeSwayOffsetCounts 10MM"=w446:refnum<vi>)
  n69 = Unbundle By Name("main ref") -> ("Config Parameters.LRMHomeSurgeOffsetCounts"=w437:refnum<vi>)
  n70 = Unbundle By Name("main ref") -> ("Config Parameters.LRMHomeSwayOffsetCounts"=w434:refnum<vi>)
  n71 = Unbundle By Name("main ref") -> ("Config Parameters.Filter%"=w433:refnum<vi>)
  n72 = Unbundle By Name("main ref") -> ("Config Parameters.Filter% 2"=w429:refnum<vi>)
  n73 = Unbundle By Name("main ref") -> ("About Screen.Temp Modbus:"=w420:refnum<vi>)
  n74 = Unbundle By Name("main ref") -> ("Config Parameters.LOAD TRIP  ENABLE"=w249:refnum<vi>)
  n75 = Unbundle By Name("main ref") -> ("Config Parameters.DEPTH TRIP VALUE"=w250:refnum<vi>)
  n76 = Unbundle By Name("main ref") -> ("Config Parameters.LOAD TRIP VALUE"=w254:refnum<vi>)
  n77 = Unbundle By Name("main ref") -> ("Config Parameters.DEPTH TRIP   ENABLE"=w255:refnum<vi>)
  n78 = Unbundle By Name("main ref") -> ("Config Parameters.CYCLIC FF TRIP VALUE"=w261:refnum<vi>)
  n79 = Unbundle By Name("main ref") -> ("Config Parameters.FF TRIP VALUE"=w262:refnum<vi>)
  n80 = Unbundle By Name("main ref") -> ("Config Parameters.CYCLIC CoF TRIP VALUE"=w267:refnum<vi>)
  n81 = Unbundle By Name("main ref") -> ("Config Parameters.CYCLIC FF TRIP  ENABLE"=w268:refnum<vi>)
  n82 = Unbundle By Name("main ref") -> ("Config Parameters.FF TRIP  ENABLE"=w276:refnum<vi>)
  n83 = Unbundle By Name("main ref") -> ("Config Parameters.COF TRIP  ENABLE"=w271:refnum<vi>)
  n84 = Unbundle By Name("main ref") -> ("Config Parameters.JOG TRIP LOAD VALUE (N)"=w120:refnum<vi>)
  n85 = Unbundle By Name("main ref") -> ("Config Parameters.CYCLIC COF TRIP  ENABLE"=w244:refnum<vi>)
  n86 = Unbundle By Name("main ref") -> ("Config Parameters.COF TRIP VALUE"=w243:refnum<vi>)
  n87 = Unbundle By Name("main ref") -> ("Config Parameters.Sway Loop Delay"=w291:refnum<vi>)
  n88 = Unbundle By Name("main ref") -> ("Config Parameters.Sway PID Speed"=w287:refnum<vi>)
  n89 = Unbundle By Name("main ref") -> ("Config Parameters.Sway Jog Speed"=w286:refnum<vi>)
  n90 = Unbundle By Name("main ref") -> ("Config Parameters.SURGE BACKWARD COUNT"=w50:refnum<vi>)
  n91 = Unbundle By Name("main ref") -> ("Config Parameters.SURGE FORWARD COUNT"=w46:refnum<vi>)
  n92 = Unbundle By Name("main ref") -> ("Config Parameters.Rotary Vertical"=w79:refnum<vi>)
  n93 = Unbundle By Name("main ref") -> ("Config Parameters.Traction"=w72:refnum<vi>)
  n94 = Unbundle By Name("main ref") -> ("Config Parameters.Scratch"=w77:refnum<vi>)
  n95 = Unbundle By Name("main ref") -> ("Config Parameters.LRM CAM"=w80:refnum<vi>)
  n96 = Unbundle By Name("main ref") -> ("Config Parameters.Sway LRM"=w85:refnum<vi>)
  n97 = Unbundle By Name("main ref") -> ("Config Parameters.Rotary Horizontal"=w68:refnum<vi>)
  n98 = Unbundle By Name("main ref") -> ("Config Parameters.SURGE SPEED"=w51:refnum<vi>)
  n99 = property class="VISAName"(reference=w5, "Value"=w1) -> (reference out=w3:refnum<vi>, error out=w4:errorcluster)  [unwired: 1 in]
  n100 = Fract/Exp String To Number(string=w413) -> (number=w391:dbl)  [unwired: 3 in, 1 out]
  n101 = Fract/Exp String To Number(string=w412) -> (number=w390:dbl)  [unwired: 3 in, 1 out]
  n102 = Fract/Exp String To Number(string=w411) -> (number=w389:dbl)  [unwired: 3 in, 1 out]
  n103 = Fract/Exp String To Number(string=w410) -> (number=w388:dbl)  [unwired: 3 in, 1 out]
  n104 = Fract/Exp String To Number(string=w409) -> (number=w387:dbl)  [unwired: 3 in, 1 out]
  n105 = Fract/Exp String To Number(string=w408) -> (number=w386:dbl)  [unwired: 3 in, 1 out]
  n106 = Fract/Exp String To Number(string=w407) -> (number=w385:dbl)  [unwired: 3 in, 1 out]
  n107 = Fract/Exp String To Number(string=w406) -> (number=w384:dbl)  [unwired: 3 in, 1 out]
  n108 = Fract/Exp String To Number(string=w405) -> (number=w383:dbl)  [unwired: 3 in, 1 out]
  n109 = Fract/Exp String To Number(string=w404) -> (number=w382:dbl)  [unwired: 3 in, 1 out]
  n110 = Fract/Exp String To Number(string=w403) -> (number=w381:dbl)  [unwired: 3 in, 1 out]
  n111 = Fract/Exp String To Number(string=w402) -> (number=w380:dbl)  [unwired: 3 in, 1 out]
  n112 = Fract/Exp String To Number(string=w401) -> (number=w379:dbl)  [unwired: 3 in, 1 out]
  n113 = Fract/Exp String To Number(string=w400) -> (number=w378:dbl)  [unwired: 3 in, 1 out]
  n114 = Fract/Exp String To Number(string=w399) -> (number=w377:dbl)  [unwired: 3 in, 1 out]
  n115 = Fract/Exp String To Number(string=w398) -> (number=w376:dbl)  [unwired: 3 in, 1 out]
  n116 = Fract/Exp String To Number(string=w397) -> (number=w375:dbl)  [unwired: 3 in, 1 out]
  n117 = Fract/Exp String To Number(string=w396) -> (number=w374:dbl)  [unwired: 3 in, 1 out]
  n118 = Fract/Exp String To Number(string=w395) -> (number=w373:dbl)  [unwired: 3 in, 1 out]
  n119 = Fract/Exp String To Number(string=w394) -> (number=w372:dbl)  [unwired: 3 in, 1 out]
  n120 = Fract/Exp String To Number(string=w393) -> (number=w371:dbl)  [unwired: 3 in, 1 out]
  n121 = Fract/Exp String To Number(string=w392) -> (number=w370:dbl)  [unwired: 3 in, 1 out]
  n122 = property class="VISAName"(reference=w420, "Value"=w415) -> (reference out=w422:refnum<vi>, error out=w421:errorcluster)  [unwired: 1 in]
  n123 = Fract/Exp String To Number(string=w353) -> (number=w366:dbl)  [unwired: 3 in, 1 out]
  n124 = Fract/Exp String To Number(string=w352) -> (number=w367:dbl)  [unwired: 3 in, 1 out]
  n125 = Fract/Exp String To Number(string=w351) -> (number=w368:dbl)  [unwired: 3 in, 1 out]
  n126 = Fract/Exp String To Number(string=w350) -> (number=w369:dbl)  [unwired: 3 in, 1 out]
  n127 = Fract/Exp String To Number(string=w116) -> (number=w117:dbl)  [unwired: 3 in, 1 out]
  n128 = Fract/Exp String To Number(string=w163) -> (number=w150:dbl)  [unwired: 3 in, 1 out]
  n129 = Fract/Exp String To Number(string=w227) -> (number=w154:dbl)  [unwired: 3 in, 1 out]
  n130 = Fract/Exp String To Number(string=w224) -> (number=w156:dbl)  [unwired: 3 in, 1 out]
  n131 = Fract/Exp String To Number(string=w226) -> (number=w146:dbl)  [unwired: 3 in, 1 out]
  n132 = Fract/Exp String To Number(string=w222) -> (number=w157:dbl)  [unwired: 3 in, 1 out]
  n133 = Fract/Exp String To Number(string=w279) -> (number=w282:dbl)  [unwired: 3 in, 1 out]
  n134 = Fract/Exp String To Number(string=w278) -> (number=w281:dbl)  [unwired: 3 in, 1 out]
  n135 = Fract/Exp String To Number(string=w277) -> (number=w280:dbl)  [unwired: 3 in, 1 out]
  n136 = property class="VISAName"(reference=w418, "Value"=w6) -> (reference out=w417:refnum<vi>, error out=w419:errorcluster)  [unwired: 1 in]
  n137 = Fract/Exp String To Number(string=w223) -> (number=w142:dbl)  [unwired: 3 in, 1 out]
  n138 = Fract/Exp String To Number(string=w42) -> (number=w54:dbl)  [unwired: 3 in, 1 out]
  n139 = property class="DigNum (strict)"(reference=w437, "Value"=w374) -> (reference out=w438:refnum<vi>, error out=w436:errorcluster)  [unwired: 1 in]
  n140 = property class="DigNum (strict)"(reference=w434, "Value"=w373) -> (reference out=w439:refnum<vi>, error out=w435:errorcluster)  [unwired: 1 in]
  n141 = property class="DigNum (strict)"(reference=w433, "Value"=w372) -> (reference out=w431:refnum<vi>, error out=w432:errorcluster)  [unwired: 1 in]
  n142 = property class="DigNum (strict)"(reference=w428, "Value"=w370) -> (reference out=w426:refnum<vi>, error out=w427:errorcluster)  [unwired: 1 in]
  n143 = property class="DigNum (strict)"(reference=w356, "Value"=w366) -> (reference out=w354:refnum<vi>, error out=w355:errorcluster)  [unwired: 1 in]
  n144 = Fract/Exp String To Number(string=w41) -> (number=w44:dbl)  [unwired: 3 in, 1 out]
  n145 = Fract/Exp String To Number(string=w40) -> (number=w43:dbl)  [unwired: 3 in, 1 out]
  n146 = property class="DigNum (strict)"(reference=w429, "Value"=w371) -> (reference out=w425:refnum<vi>, error out=w430:errorcluster)  [unwired: 1 in]
  n147 = property class="DigNum (strict)"(reference=w357, "Value"=w367) -> (reference out=w359:refnum<vi>, error out=w358:errorcluster)  [unwired: 1 in]
  n148 = property class="DigNum (strict)"(reference=w362, "Value"=w369) -> (reference out=w364:refnum<vi>, error out=w363:errorcluster)  [unwired: 1 in]
  n149 = property class="DigNum (strict)"(reference=w120, "Value"=w117) -> (reference out=w118:refnum<vi>, error out=w119:errorcluster)  [unwired: 1 in]
  n150 = property class="DigNum (strict)"(reference=w453, "Value"=w379) -> (reference out=w452:refnum<vi>, error out=w454:errorcluster)  [unwired: 1 in]
  n151 = property class="DigNum (strict)"(reference=w443, "Value"=w376) -> (reference out=w441:refnum<vi>, error out=w444:errorcluster)  [unwired: 1 in]
  n152 = property class="DigNum (strict)"(reference=w446, "Value"=w375) -> (reference out=w440:refnum<vi>, error out=w445:errorcluster)  [unwired: 1 in]
  n153 = property class="DigNum (strict)"(reference=w361, "Value"=w368) -> (reference out=w365:refnum<vi>, error out=w360:errorcluster)  [unwired: 1 in]
  n154 = property class="DigNum (strict)"(reference=w489, "Value"=w391) -> (reference out=w487:refnum<vi>, error out=w488:errorcluster)  [unwired: 1 in]
  n155 = property class="DigNum (strict)"(reference=w467, "Value"=w385) -> (reference out=w424:refnum<vi>, error out=w468:errorcluster)  [unwired: 1 in]
  n156 = property class="DigNum (strict)"(reference=w450, "Value"=w378) -> (reference out=w451:refnum<vi>, error out=w449:errorcluster)  [unwired: 1 in]
  n157 = property class="DigNum (strict)"(reference=w447, "Value"=w377) -> (reference out=w442:refnum<vi>, error out=w448:errorcluster)  [unwired: 1 in]
  n158 = property class="DigNum (strict)"(reference=w484, "Value"=w390) -> (reference out=w486:refnum<vi>, error out=w485:errorcluster)  [unwired: 1 in]
  n159 = property class="DigNum (strict)"(reference=w478, "Value"=w389) -> (reference out=w480:refnum<vi>, error out=w479:errorcluster)  [unwired: 1 in]
  n160 = property class="DigNum (strict)"(reference=w477, "Value"=w387) -> (reference out=w472:refnum<vi>, error out=w476:errorcluster)  [unwired: 1 in]
  n161 = property class="DigNum (strict)"(reference=w471, "Value"=w384) -> (reference out=w469:refnum<vi>, error out=w470:errorcluster)  [unwired: 1 in]
  n162 = property class="DigNum (strict)"(reference=w465, "Value"=w383) -> (reference out=w464:refnum<vi>, error out=w466:errorcluster)  [unwired: 1 in]
  n163 = property class="DigNum (strict)"(reference=w462, "Value"=w382) -> (reference out=w463:refnum<vi>, error out=w461:errorcluster)  [unwired: 1 in]
  n164 = property class="DigNum (strict)"(reference=w459, "Value"=w381) -> (reference out=w458:refnum<vi>, error out=w460:errorcluster)  [unwired: 1 in]
  n165 = property class="DigNum (strict)"(reference=w456, "Value"=w380) -> (reference out=w457:refnum<vi>, error out=w455:errorcluster)  [unwired: 1 in]
  n166 = property class="DigNum (strict)"(reference=w483, "Value"=w388) -> (reference out=w481:refnum<vi>, error out=w482:errorcluster)  [unwired: 1 in]
  n167 = property class="DigNum (strict)"(reference=w473, "Value"=w386) -> (reference out=w475:refnum<vi>, error out=w474:errorcluster)  [unwired: 1 in]
  n168 = property class="DigNum (strict)"(reference=w291, "Value"=w282) -> (reference out=w289:refnum<vi>, error out=w290:errorcluster)  [unwired: 1 in]
  n169 = property class="DigNum (strict)"(reference=w286, "Value"=w280) -> (reference out=w284:refnum<vi>, error out=w285:errorcluster)  [unwired: 1 in]
  n170 = property class="DigNum (strict)"(reference=w250, "Value"=w154) -> (reference out=w252:refnum<vi>, error out=w251:errorcluster)  [unwired: 1 in]
  n171 = property class="DigNum (strict)"(reference=w261, "Value"=w156) -> (reference out=w259:refnum<vi>, error out=w260:errorcluster)  [unwired: 1 in]
  n172 = property class="DigNum (strict)"(reference=w262, "Value"=w142) -> (reference out=w264:refnum<vi>, error out=w263:errorcluster)  [unwired: 1 in]
  n173 = property class="DigNum (strict)"(reference=w267, "Value"=w157) -> (reference out=w265:refnum<vi>, error out=w266:errorcluster)  [unwired: 1 in]
  n174 = property class="DigNum (strict)"(reference=w287, "Value"=w281) -> (reference out=w283:refnum<vi>, error out=w288:errorcluster)  [unwired: 1 in]
  n175 = property class="DigNum (strict)"(reference=w254, "Value"=w146) -> (reference out=w258:refnum<vi>, error out=w253:errorcluster)  [unwired: 1 in]
  n176 = property class="Bool (strict)"(reference=w244, "Value"=w162) -> (reference out=w246:refnum<vi>, error out=w245:errorcluster)  [unwired: 1 in]
  n177 = property class="Bool (strict)"(reference=w85, "Value"=w111) -> (reference out=w83:refnum<vi>, error out=w84:errorcluster)  [unwired: 1 in]
  n178 = property class="DigNum (strict)"(reference=w243, "Value"=w150) -> (reference out=w241:refnum<vi>, error out=w242:errorcluster)  [unwired: 1 in]
  n179 = property class="DigNum (strict)"(reference=w51, "Value"=w54) -> (reference out=w53:refnum<vi>, error out=w52:errorcluster)  [unwired: 1 in]
  n180 = property class="Bool (strict)"(reference=w255, "Value"=w155) -> (reference out=w257:refnum<vi>, error out=w256:errorcluster)  [unwired: 1 in]
  n181 = property class="Bool (strict)"(reference=w268, "Value"=w158) -> (reference out=w270:refnum<vi>, error out=w269:errorcluster)  [unwired: 1 in]
  n182 = property class="Bool (strict)"(reference=w276, "Value"=w159) -> (reference out=w274:refnum<vi>, error out=w275:errorcluster)  [unwired: 1 in]
  n183 = property class="Bool (strict)"(reference=w271, "Value"=w160) -> (reference out=w273:refnum<vi>, error out=w272:errorcluster)  [unwired: 1 in]
  n184 = property class="Bool (strict)"(reference=w249, "Value"=w161) -> (reference out=w247:refnum<vi>, error out=w248:errorcluster)  [unwired: 1 in]
  n185 = property class="Bool (strict)"(reference=w79, "Value"=w115) -> (reference out=w71:refnum<vi>, error out=w78:errorcluster)  [unwired: 1 in]
  n186 = property class="Bool (strict)"(reference=w72, "Value"=w114) -> (reference out=w74:refnum<vi>, error out=w73:errorcluster)  [unwired: 1 in]
  n187 = property class="Bool (strict)"(reference=w77, "Value"=w113) -> (reference out=w75:refnum<vi>, error out=w76:errorcluster)  [unwired: 1 in]
  n188 = property class="Bool (strict)"(reference=w80, "Value"=w112) -> (reference out=w82:refnum<vi>, error out=w81:errorcluster)  [unwired: 1 in]
  n189 = property class="Bool (strict)"(reference=w68, "Value"=w62) -> (reference out=w70:refnum<vi>, error out=w69:errorcluster)  [unwired: 1 in]
  n190 = property class="DigNum (strict)"(reference=w50, "Value"=w44) -> (reference out=w48:refnum<vi>, error out=w49:errorcluster)  [unwired: 1 in]
  n191 = property class="DigNum (strict)"(reference=w46, "Value"=w43) -> (reference out=w45:refnum<vi>, error out=w47:errorcluster)  [unwired: 1 in]
  n192 = Close Reference(reference=w3, error in (no error)=w4) -> ()  [unwired: 1 out]
  n193 = Close Reference(reference=w422, error in (no error)=w421) -> ()  [unwired: 1 out]
  n194 = Close Reference(reference=w417, error in (no error)=w419) -> ()  [unwired: 1 out]
  n195 = Close Reference(reference=w438, error in (no error)=w436) -> ()  [unwired: 1 out]
  n196 = Close Reference(reference=w439, error in (no error)=w435) -> ()  [unwired: 1 out]
  n197 = Close Reference(reference=w431, error in (no error)=w432) -> ()  [unwired: 1 out]
  n198 = Close Reference(reference=w426, error in (no error)=w427) -> ()  [unwired: 1 out]
  n199 = Close Reference(reference=w354, error in (no error)=w355) -> ()  [unwired: 1 out]
  n200 = Close Reference(reference=w425, error in (no error)=w430) -> ()  [unwired: 1 out]
  n201 = Close Reference(reference=w359, error in (no error)=w358) -> ()  [unwired: 1 out]
  n202 = Close Reference(reference=w364, error in (no error)=w363) -> ()  [unwired: 1 out]
  n203 = Close Reference(reference=w118, error in (no error)=w119) -> ()  [unwired: 1 out]
  n204 = Close Reference(reference=w452, error in (no error)=w454) -> ()  [unwired: 1 out]
  n205 = Close Reference(reference=w441, error in (no error)=w444) -> ()  [unwired: 1 out]
  n206 = Close Reference(reference=w440, error in (no error)=w445) -> ()  [unwired: 1 out]
  n207 = Close Reference(reference=w365, error in (no error)=w360) -> ()  [unwired: 1 out]
  n208 = Close Reference(reference=w487, error in (no error)=w488) -> ()  [unwired: 1 out]
  n209 = Close Reference(reference=w424, error in (no error)=w468) -> ()  [unwired: 1 out]
  n210 = Close Reference(reference=w451, error in (no error)=w449) -> ()  [unwired: 1 out]
  n211 = Close Reference(reference=w442, error in (no error)=w448) -> ()  [unwired: 1 out]
  n212 = Close Reference(reference=w486, error in (no error)=w485) -> ()  [unwired: 1 out]
  n213 = Close Reference(reference=w480, error in (no error)=w479) -> ()  [unwired: 1 out]
  n214 = Close Reference(reference=w472, error in (no error)=w476) -> ()  [unwired: 1 out]
  n215 = Close Reference(reference=w469, error in (no error)=w470) -> ()  [unwired: 1 out]
  n216 = Close Reference(reference=w464, error in (no error)=w466) -> ()  [unwired: 1 out]
  n217 = Close Reference(reference=w463, error in (no error)=w461) -> ()  [unwired: 1 out]
  n218 = Close Reference(reference=w458, error in (no error)=w460) -> ()  [unwired: 1 out]
  n219 = Close Reference(reference=w457, error in (no error)=w455) -> ()  [unwired: 1 out]
  n220 = Close Reference(reference=w481, error in (no error)=w482) -> ()  [unwired: 1 out]
  n221 = Close Reference(reference=w475, error in (no error)=w474) -> ()  [unwired: 1 out]
  n222 = Close Reference(reference=w246, error in (no error)=w245) -> ()  [unwired: 1 out]
  n223 = Close Reference(reference=w83, error in (no error)=w84) -> ()  [unwired: 1 out]
  n224 = Close Reference(reference=w289, error in (no error)=w290) -> ()  [unwired: 1 out]
  n225 = Close Reference(reference=w284, error in (no error)=w285) -> ()  [unwired: 1 out]
  n226 = Close Reference(reference=w252, error in (no error)=w251) -> ()  [unwired: 1 out]
  n227 = Close Reference(reference=w257, error in (no error)=w256) -> ()  [unwired: 1 out]
  n228 = Close Reference(reference=w259, error in (no error)=w260) -> ()  [unwired: 1 out]
  n229 = Close Reference(reference=w264, error in (no error)=w263) -> ()  [unwired: 1 out]
  n230 = Close Reference(reference=w265, error in (no error)=w266) -> ()  [unwired: 1 out]
  n231 = Close Reference(reference=w270, error in (no error)=w269) -> ()  [unwired: 1 out]
  n232 = Close Reference(reference=w274, error in (no error)=w275) -> ()  [unwired: 1 out]
  n233 = Close Reference(reference=w273, error in (no error)=w272) -> ()  [unwired: 1 out]
  n234 = Close Reference(reference=w247, error in (no error)=w248) -> ()  [unwired: 1 out]
  n235 = Close Reference(reference=w71, error in (no error)=w78) -> ()  [unwired: 1 out]
  n236 = Close Reference(reference=w74, error in (no error)=w73) -> ()  [unwired: 1 out]
  n237 = Close Reference(reference=w75, error in (no error)=w76) -> ()  [unwired: 1 out]
  n238 = Close Reference(reference=w82, error in (no error)=w81) -> ()  [unwired: 1 out]
  n239 = Close Reference(reference=w70, error in (no error)=w69) -> ()  [unwired: 1 out]
  n240 = Close Reference(reference=w283, error in (no error)=w288) -> ()  [unwired: 1 out]
  n241 = Close Reference(reference=w258, error in (no error)=w253) -> ()  [unwired: 1 out]
  n242 = Close Reference(reference=w241, error in (no error)=w242) -> ()  [unwired: 1 out]
  n243 = Close Reference(reference=w53, error in (no error)=w52) -> ()  [unwired: 1 out]
  n244 = Close Reference(reference=w48, error in (no error)=w49) -> ()  [unwired: 1 out]
  n245 = Close Reference(reference=w45, error in (no error)=w47) -> ()  [unwired: 1 out]
  n246 = for {
    tunnel: "NEW PID PARAMETERS" ("WRITE /READ SECTION") -> [w521]
    tunnel: [w520] -> w38
    tunnel: string[] ["PID DELAY (sec)", "Kp", "Ki", "Kd", "Deaadband", "pct_scale", "Init_step", "i_limit", "Max Step Limit", "Min_pos_limit", "Max_pos_limit", "Fine_tune_zone", "min_deadband_floor", "min_finetune_floor", "dynamic_spindle_noise_scalar", "filter_alpha"] -> [w517] mode=indexing
    tunnel: [w516] -> w321 mode=indexing
    tunnel: w348 -> [w515]
    n247 = call "CONFIG FILE MAIN Unitest.vi"("WRITE /READ SECTION"=w521, "READ KEY"=w517, "error in"=w515, "PARAMETER/CONFIG"=TRUE, "Config Enum"=Config_file__FGV_Unitest_enum."READ") -> ("READ VALUE"=w516:string, "error out"=w520:errorcluster)  [unwired: 13 in]
  }
  n248 = Unbundle By Name("main ref") -> ("Loading.Enter the CoF Trip"=w153:refnum<vi>)
  n249 = Unbundle By Name("main ref") -> ("Main Screen.Load Disable Trip"=w191:refnum<vi>)
  n250 = Unbundle By Name("main ref") -> ("Main Screen.FF Disable Trip"=w164:refnum<vi>)
  n251 = Unbundle By Name("main ref") -> ("Main Screen.COF Disable Trip"=w169:refnum<vi>)
  n252 = Unbundle By Name("main ref") -> ("Main Screen.Cyclic FF Disable Trip"=w172:refnum<vi>)
  n253 = Unbundle By Name("main ref") -> ("Main Screen.cyclic COF Disable Trip"=w196:refnum<vi>)
  n254 = Unbundle By Name("main ref") -> ("Main Screen.FF TRIP"=w178:refnum<vi>)
  n255 = Unbundle By Name("main ref") -> ("Main Screen.COF TRIP"=w197:refnum<vi>)
  n256 = Unbundle By Name("main ref") -> ("Main Screen.Depth Trip"=w190:refnum<vi>)
  n257 = Unbundle By Name("main ref") -> ("Main Screen.Depth Trip 2"=w185:refnum<vi>)
  n258 = Unbundle By Name("main ref") -> ("Main Screen.Cyclic FF TRIP"=w179:refnum<vi>)
  n259 = Unbundle By Name("main ref") -> ("Main Screen.cyclic COF TRIP"=w173:refnum<vi>)
  n260 = Unbundle By Name("main ref") -> ("Main Screen.NL Trip 2"=w186:refnum<vi>)
  n261 = Unbundle By Name("main ref") -> ("New PID LOGIC.PID SDelay"=w345:refnum<vi>)
  n262 = Unbundle By Name("main ref") -> ("New PID LOGIC.Kp"=w344:refnum<vi>)
  n263 = Unbundle By Name("main ref") -> ("New PID LOGIC.Ki"=w339:refnum<vi>)
  n264 = Unbundle By Name("main ref") -> ("New PID LOGIC.Kd"=w338:refnum<vi>)
  n265 = Unbundle By Name("main ref") -> ("New PID LOGIC.Deadband"=w334:refnum<vi>)
  n266 = Unbundle By Name("main ref") -> ("New PID LOGIC.pct_scale"=w333:refnum<vi>)
  n267 = Unbundle By Name("main ref") -> ("New PID LOGIC.Init Step"=w330:refnum<vi>)
  n268 = Unbundle By Name("main ref") -> ("New PID LOGIC.i_limit"=w329:refnum<vi>)
  n269 = Unbundle By Name("main ref") -> ("New PID LOGIC.Max Step Linit"=w326:refnum<vi>)
  n270 = Unbundle By Name("main ref") -> ("New PID LOGIC.Max_pos_limit"=w324:refnum<vi>)
  n271 = Unbundle By Name("main ref") -> ("New PID LOGIC.Min_pos_limit"=w323:refnum<vi>)
  n272 = Unbundle By Name("main ref") -> ("New PID LOGIC.min_deadband_floor"=w141:refnum<vi>)
  n273 = Unbundle By Name("main ref") -> ("New PID LOGIC.min_finetune_floor"=w138:refnum<vi>)
  n274 = Unbundle By Name("main ref") -> ("New PID LOGIC.dynamic_spindle_noise_scalar"=w136:refnum<vi>)
  n275 = Unbundle By Name("main ref") -> ("New PID LOGIC.filter_alpha"=w135:refnum<vi>)
  n276 = Index Array(array=w321) -> (element #1=w320:string, element #2=w319:string, element #3=w316:string, element #4=w315:string, element #5=w314:string, element #6=w313:string, element #7=w308:string, element #8=w307:string, element #9=w306:string, element #10=w305:string, element #11=w304:string, element #12=w126:string, element #13=w125:string, element #14=w124:string, element #15=w123:string)  [unwired: 15 in]
  n277 = property class="DigNum (strict)"(reference=w153, "Value"=w150) -> (reference out=w151:refnum<vi>, error out=w152:errorcluster)  [unwired: 1 in]
  n278 = property class="DigNum (strict)"(reference=w190, "Value"=w154) -> (reference out=w188:refnum<vi>, error out=w189:errorcluster)  [unwired: 1 in]
  n279 = property class="DigNum (strict)"(reference=w179, "Value"=w156) -> (reference out=w181:refnum<vi>, error out=w180:errorcluster)  [unwired: 1 in]
  n280 = property class="DigNum (strict)"(reference=w178, "Value"=w142) -> (reference out=w176:refnum<vi>, error out=w177:errorcluster)  [unwired: 1 in]
  n281 = property class="DigNum (strict)"(reference=w173, "Value"=w157) -> (reference out=w175:refnum<vi>, error out=w174:errorcluster)  [unwired: 1 in]
  n282 = property class="DigNum (strict)"(reference=w186, "Value"=w146) -> (reference out=w182:refnum<vi>, error out=w187:errorcluster)  [unwired: 1 in]
  n283 = property class="Bool (strict)"(reference=w196, "Value"=w162) -> (reference out=w194:refnum<vi>, error out=w195:errorcluster)  [unwired: 1 in]
  n284 = property class="DigNum (strict)"(reference=w197, "Value"=w150) -> (reference out=w199:refnum<vi>, error out=w198:errorcluster)  [unwired: 1 in]
  n285 = property class="Bool (strict)"(reference=w185, "Value"=w155) -> (reference out=w183:refnum<vi>, error out=w184:errorcluster)  [unwired: 1 in]
  n286 = property class="Bool (strict)"(reference=w172, "Value"=w158) -> (reference out=w170:refnum<vi>, error out=w171:errorcluster)  [unwired: 1 in]
  n287 = property class="Bool (strict)"(reference=w164, "Value"=w159) -> (reference out=w166:refnum<vi>, error out=w165:errorcluster)  [unwired: 1 in]
  n288 = property class="Bool (strict)"(reference=w169, "Value"=w160) -> (reference out=w167:refnum<vi>, error out=w168:errorcluster)  [unwired: 1 in]
  n289 = property class="Bool (strict)"(reference=w191, "Value"=w161) -> (reference out=w193:refnum<vi>, error out=w192:errorcluster)  [unwired: 1 in]
  n290 = Unbundle By Name("main ref") -> ("Loading.Enter the Normal load Trip"=w149:refnum<vi>)
  n291 = Fract/Exp String To Number(string=w320) -> (number=w318:dbl)  [unwired: 3 in, 1 out]
  n292 = Fract/Exp String To Number(string=w319) -> (number=w317:dbl)  [unwired: 3 in, 1 out]
  n293 = Fract/Exp String To Number(string=w316) -> (number=w312:dbl)  [unwired: 3 in, 1 out]
  n294 = Fract/Exp String To Number(string=w126) -> (number=w133:dbl)  [unwired: 3 in, 1 out]
  n295 = Fract/Exp String To Number(string=w125) -> (number=w132:dbl)  [unwired: 3 in, 1 out]
  n296 = Fract/Exp String To Number(string=w124) -> (number=w131:dbl)  [unwired: 3 in, 1 out]
  n297 = Fract/Exp String To Number(string=w123) -> (number=w130:dbl)  [unwired: 3 in, 1 out]
  n298 = Close Reference(reference=w151, error in (no error)=w152) -> ()  [unwired: 1 out]
  n299 = Fract/Exp String To Number(string=w315) -> (number=w311:dbl)  [unwired: 3 in, 1 out]
  n300 = Fract/Exp String To Number(string=w314) -> (number=w310:dbl)  [unwired: 3 in, 1 out]
  n301 = Fract/Exp String To Number(string=w313) -> (number=w309:dbl)  [unwired: 3 in, 1 out]
  n302 = Fract/Exp String To Number(string=w308) -> (number=w303:dbl)  [unwired: 3 in, 1 out]
  n303 = Fract/Exp String To Number(string=w307) -> (number=w302:dbl)  [unwired: 3 in, 1 out]
  n304 = Fract/Exp String To Number(string=w306) -> (number=w301:dbl)  [unwired: 3 in, 1 out]
  n305 = Fract/Exp String To Number(string=w305) -> (number=w300:dbl)  [unwired: 3 in, 1 out]
  n306 = Fract/Exp String To Number(string=w304) -> (number=w299:dbl)  [unwired: 3 in, 1 out]
  n307 = Close Reference(reference=w194, error in (no error)=w195) -> ()  [unwired: 1 out]
  n308 = Unbundle By Name("main ref") -> ("Loading.Enter the Friction Force Trip"=w145:refnum<vi>)
  n309 = Close Reference(reference=w188, error in (no error)=w189) -> ()  [unwired: 1 out]
  n310 = Close Reference(reference=w183, error in (no error)=w184) -> ()  [unwired: 1 out]
  n311 = Close Reference(reference=w181, error in (no error)=w180) -> ()  [unwired: 1 out]
  n312 = Close Reference(reference=w176, error in (no error)=w177) -> ()  [unwired: 1 out]
  n313 = Close Reference(reference=w175, error in (no error)=w174) -> ()  [unwired: 1 out]
  n314 = Close Reference(reference=w170, error in (no error)=w171) -> ()  [unwired: 1 out]
  n315 = Close Reference(reference=w166, error in (no error)=w165) -> ()  [unwired: 1 out]
  n316 = Close Reference(reference=w167, error in (no error)=w168) -> ()  [unwired: 1 out]
  n317 = Close Reference(reference=w193, error in (no error)=w192) -> ()  [unwired: 1 out]
  n318 = Close Reference(reference=w182, error in (no error)=w187) -> ()  [unwired: 1 out]
  n319 = Close Reference(reference=w199, error in (no error)=w198) -> ()  [unwired: 1 out]
  n320 = property class="DigNum (strict)"(reference=w345, "Value"=w318) -> (reference out=w347:refnum<vi>, error out=w346:errorcluster)  [unwired: 1 in]
  n321 = property class="DigNum (strict)"(reference=w344, "Value"=w317) -> (reference out=w342:refnum<vi>, error out=w343:errorcluster)  [unwired: 1 in]
  n322 = property class="DigNum (strict)"(reference=w339, "Value"=w312) -> (reference out=w341:refnum<vi>, error out=w340:errorcluster)  [unwired: 1 in]
  n323 = property class="DigNum (strict)"(reference=w141, "Value"=w133) -> (reference out=w122:refnum<vi>, error out=w140:errorcluster)  [unwired: 1 in]
  n324 = property class="DigNum (strict)"(reference=w138, "Value"=w132) -> (reference out=w129:refnum<vi>, error out=w139:errorcluster)  [unwired: 1 in]
  n325 = property class="DigNum (strict)"(reference=w136, "Value"=w131) -> (reference out=w128:refnum<vi>, error out=w137:errorcluster)  [unwired: 1 in]
  n326 = property class="DigNum (strict)"(reference=w135, "Value"=w130) -> (reference out=w127:refnum<vi>, error out=w134:errorcluster)  [unwired: 1 in]
  n327 = property class="DigNum (strict)"(reference=w338, "Value"=w311) -> (reference out=w336:refnum<vi>, error out=w337:errorcluster)  [unwired: 1 in]
  n328 = property class="DigNum (strict)"(reference=w334, "Value"=w310) -> (reference out=w297:refnum<vi>, error out=w335:errorcluster)  [unwired: 1 in]
  n329 = property class="DigNum (strict)"(reference=w333, "Value"=w309) -> (reference out=w298:refnum<vi>, error out=w332:errorcluster)  [unwired: 1 in]
  n330 = property class="DigNum (strict)"(reference=w330, "Value"=w303) -> (reference out=w296:refnum<vi>, error out=w331:errorcluster)  [unwired: 1 in]
  n331 = property class="DigNum (strict)"(reference=w329, "Value"=w302) -> (reference out=w295:refnum<vi>, error out=w328:errorcluster)  [unwired: 1 in]
  n332 = property class="DigNum (strict)"(reference=w326, "Value"=w301) -> (reference out=w294:refnum<vi>, error out=w327:errorcluster)  [unwired: 1 in]
  n333 = property class="DigNum (strict)"(reference=w324, "Value"=w300) -> (reference out=w293:refnum<vi>, error out=w325:errorcluster)  [unwired: 1 in]
  n334 = property class="DigNum (strict)"(reference=w323, "Value"=w299) -> (reference out=w292:refnum<vi>, error out=w322:errorcluster)  [unwired: 1 in]
  n335 = property class="DigNum (strict)"(reference=w149, "Value"=w146) -> (reference out=w147:refnum<vi>, error out=w148:errorcluster)  [unwired: 1 in]
  n336 = property class="DigNum (strict)"(reference=w145, "Value"=w142) -> (reference out=w143:refnum<vi>, error out=w144:errorcluster)  [unwired: 1 in]
  n337 = Close Reference(reference=w347, error in (no error)=w346) -> ()  [unwired: 1 out]
  n338 = Close Reference(reference=w342, error in (no error)=w343) -> ()  [unwired: 1 out]
  n339 = Close Reference(reference=w341, error in (no error)=w340) -> ()  [unwired: 1 out]
  n340 = Close Reference(reference=w122, error in (no error)=w140) -> ()  [unwired: 1 out]
  n341 = Close Reference(reference=w129, error in (no error)=w139) -> ()  [unwired: 1 out]
  n342 = Close Reference(reference=w128, error in (no error)=w137) -> ()  [unwired: 1 out]
  n343 = Close Reference(reference=w127, error in (no error)=w134) -> ()  [unwired: 1 out]
  n344 = Close Reference(reference=w336, error in (no error)=w337) -> ()  [unwired: 1 out]
  n345 = Close Reference(reference=w297, error in (no error)=w335) -> ()  [unwired: 1 out]
  n346 = Close Reference(reference=w298, error in (no error)=w332) -> ()  [unwired: 1 out]
  n347 = Close Reference(reference=w296, error in (no error)=w331) -> ()  [unwired: 1 out]
  n348 = Close Reference(reference=w295, error in (no error)=w328) -> ()  [unwired: 1 out]
  n349 = Close Reference(reference=w294, error in (no error)=w327) -> ()  [unwired: 1 out]
  n350 = Close Reference(reference=w293, error in (no error)=w325) -> ()  [unwired: 1 out]
  n351 = Close Reference(reference=w292, error in (no error)=w322) -> ()  [unwired: 1 out]
  n352 = Close Reference(reference=w147, error in (no error)=w148) -> ()  [unwired: 1 out]
  n353 = Close Reference(reference=w143, error in (no error)=w144) -> ()  [unwired: 1 out]
  n354 = for {
    tunnel: "ABOUT SCREEN" ("WRITE /READ SECTION") -> [w528]
    tunnel: [w527] -> w37
    tunnel: string[] ["version", "Operating System", "Version", "Workorder", "runtime", "Instrument Serial Number", "Firmware version"] -> [w524] mode=indexing
    tunnel: [w523] -> w35 mode=indexing
    tunnel: w38 -> [w522]
    n355 = call "CONFIG FILE MAIN Unitest.vi"("WRITE /READ SECTION"=w528, "READ KEY"=w524, "error in"=w522, "PARAMETER/CONFIG"=TRUE, "Config Enum"=Config_file__FGV_Unitest_enum."READ") -> ("READ VALUE"=w523:string, "error out"=w527:errorcluster)  [unwired: 13 in]
  }
  n356 = Index Array(array=w35) -> (element #1=w25:string, element #2=w15:string, element #3=w14:string, element #4=w13:string, element #5=w12:string, element #6=w11:string, element #7=w7:string)  [unwired: 7 in]
  n357 = call "CONFIG FILE MAIN Unitest.vi"("error in"=w37, "Config Enum"=Config_file__FGV_Unitest_enum."CLOSE") -> ("error out"=→"error out":errorcluster)  [unwired: 16 in, 1 out]
  n358 = Unbundle By Name("main ref") -> ("ABOUT.Operating System"=w29:refnum<vi>)
  n359 = Unbundle By Name("main ref") -> ("ABOUT.Instrument Serial"=w22:refnum<vi>)
  n360 = Unbundle By Name("main ref") -> ("ABOUT.Firmware Version"=w8:refnum<vi>)
  n361 = Unbundle By Name("main ref") -> ("ABOUT.Workorder"=w16:refnum<vi>)
  n362 = Unbundle By Name("main ref") -> ("ABOUT.version"=w34:refnum<vi>)
  n363 = Unbundle By Name("main ref") -> ("ABOUT.Version"=w28:refnum<vi>)
  n364 = Unbundle By Name("main ref") -> ("ABOUT.Runtime"=w21:refnum<vi>)
  n365 = property class="Str"(reference=w34, "Value"=w25) -> (reference out=w32:refnum<vi>, error out=w33:errorcluster)  [unwired: 1 in]
  n366 = property class="Str"(reference=w29, "Value"=w15) -> (reference out=w31:refnum<vi>, error out=w30:errorcluster)  [unwired: 1 in]
  n367 = property class="Str"(reference=w28, "Value"=w14) -> (reference out=w26:refnum<vi>, error out=w27:errorcluster)  [unwired: 1 in]
  n368 = property class="Str"(reference=w16, "Value"=w13) -> (reference out=w18:refnum<vi>, error out=w17:errorcluster)  [unwired: 1 in]
  n369 = property class="Str"(reference=w21, "Value"=w12) -> (reference out=w19:refnum<vi>, error out=w20:errorcluster)  [unwired: 1 in]
  n370 = property class="Str"(reference=w22, "Value"=w11) -> (reference out=w24:refnum<vi>, error out=w23:errorcluster)  [unwired: 1 in]
  n371 = property class="Str"(reference=w8, "Value"=w7) -> (reference out=w10:refnum<vi>, error out=w9:errorcluster)  [unwired: 1 in]
  n372 = Close Reference(reference=w32, error in (no error)=w33) -> ()  [unwired: 1 out]
  n373 = Close Reference(reference=w31, error in (no error)=w30) -> ()  [unwired: 1 out]
  n374 = Close Reference(reference=w26, error in (no error)=w27) -> ()  [unwired: 1 out]
  n375 = Close Reference(reference=w18, error in (no error)=w17) -> ()  [unwired: 1 out]
  n376 = Close Reference(reference=w19, error in (no error)=w20) -> ()  [unwired: 1 out]
  n377 = Close Reference(reference=w24, error in (no error)=w23) -> ()  [unwired: 1 out]
  n378 = Close Reference(reference=w10, error in (no error)=w9) -> ()  [unwired: 1 out]
